vi "OAT Orbit Plot (Filtered).vi"(0 "magnitudes":T5(array[cluster]) {"magnitude" format="%.2f"; "time/rev/rpm" format="%.2f"}, 1 "orbit plot ref":refnum<vi>, 2 "reset? (F)":bool, 3 "order to display":dbl=1.0 format="%.2f", 5 "phases [phase lag]":cluster{"time/rev/rpm":dbl[], "phase":dbl[]}[](array[cluster]) {"phase" format="%.2f"; "time/rev/rpm" format="%.2f"}, 7 "magnitude/phase position info":T1, 9 "revolutions to display [rev]":cluster{"start":dbl, "duration":dbl}={"start"=0.0, "duration"=1.0} {"duration" format="%.2f"; "start" format="%.2f"}, 11 "error in (no error)":errorcluster, 12 "channel settings":T2={"shaft rotating direction"=0, "probe angles [deg]"={"X"=0, "Y"=90}} {"probe angles [deg]"."Y" max=360 step=1; "probe angles [deg]"."X" max=360 step=1; "shaft rotating direction" items=["CCW", "CW"]}, 13 "view info":T4={"dB on? (F)"=FALSE, "unwrap phase? (T)"=TRUE, "unit in degree? (T)"=TRUE}, 14 "samples/rev wanted":i32=64) -> (4 "orbit plot":T3, 10 "orbit precession direction":u16(ring) items=["forward", "backward"], 15 "error out":errorcluster)   [LabVIEW 2017]
doc: "Draws an orbit plot with unfiltered or filtered data on an XY graph. The unfiltered data comes from the <B>even-angle signals</B> input, and the filtered data comes from the <B>magnitudes</B> and <B>phases [phase lag]</B> inputs."
uses:
  <vilib>/addons/Sound and Vibration/Order Analysis/Backward Compatibility/SubVIs/oa_Orbit Plot Control.ctl
  <vilib>/addons/Sound and Vibration/Order Analysis/Misc/OAT Position Info.ctl
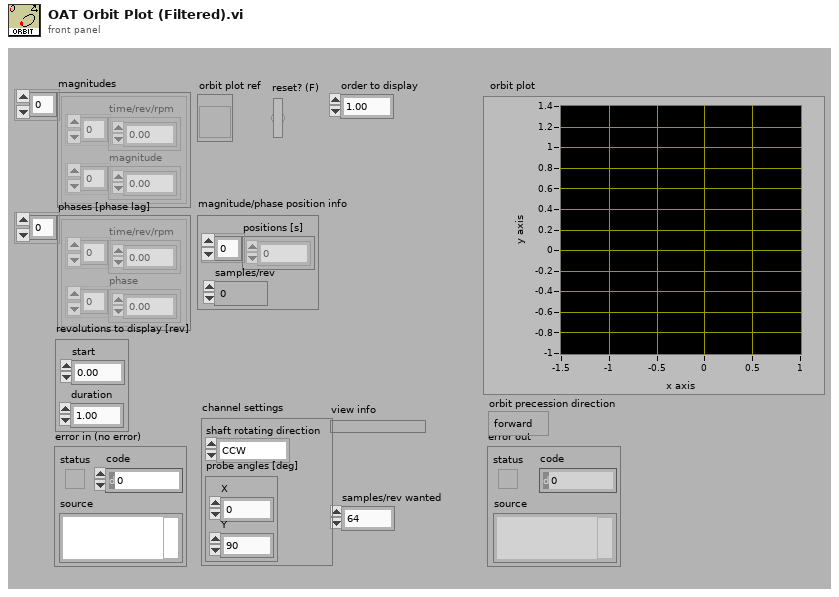
[diagram p1: front panel]
types:
  T1 = typedef "OAT Position Info.ctl" = cluster{"positions [s]":dbl[], "samples/rev":dbl}
  T2 = cluster{"shaft rotating direction":u16, "probe angles [deg]":cluster{"X":u32, "Y":u32}}
  T3 = typedef "oa_Orbit Plot Control.ctl" = cluster{dbl[], dbl[]}[]
  T4 = cluster{"dB on? (F)":bool, "unwrap phase? (T)":bool, "unit in degree? (T)":bool}
  T5 = cluster{"time/rev/rpm":dbl[], "magnitude":dbl[]}[]
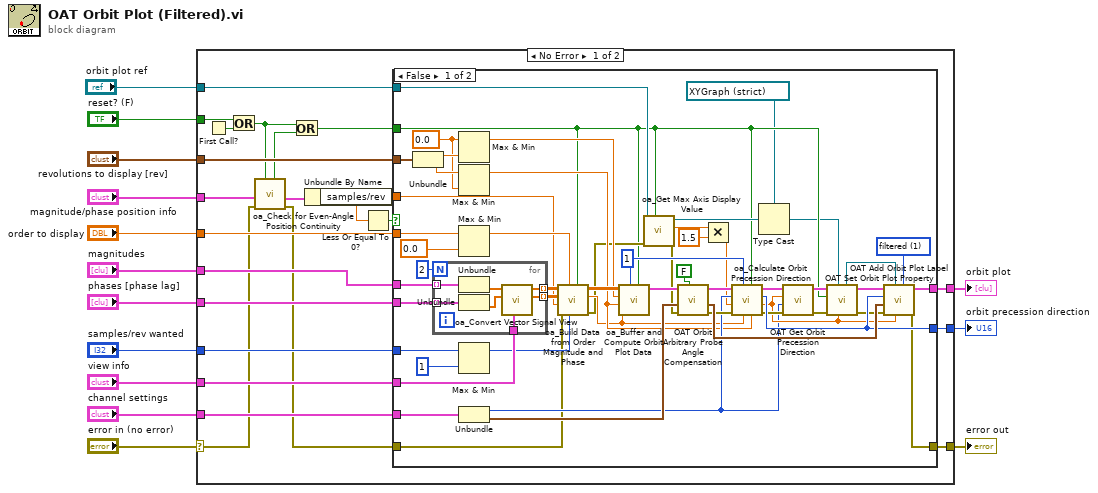
[diagram p0: block diagram]
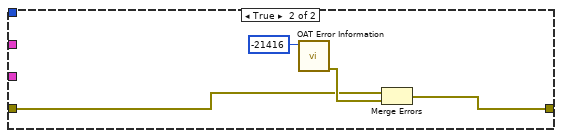
[diagram p2: hidden frame]
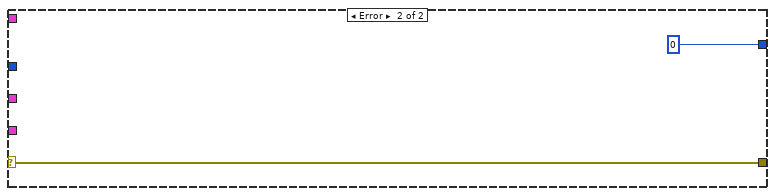
[diagram p3: hidden frame]
diagram:
  n1 = case shown="No Error" "error in (no error)" {
    selector: "error in (no error)" -> [w16 w102]
    tunnel: "order to display" -> [w27 _]
    tunnel: "magnitudes" -> [w36 _]
    tunnel: "phases [phase lag]" -> [w35 _]
    tunnel: "view info" -> [w28 _]
    tunnel: "revolutions to display [rev]" -> [w34 _]
    tunnel: [w33 _] -> w6
    tunnel: [w29 w102] -> w9
    tunnel: [w30 u16 0 ("orbit precession direction")] -> w8
    tunnel: "samples/rev wanted" -> [w32 _]
    tunnel: "channel settings" -> [w31 _]
    tunnel: "magnitude/phase position info" -> [w21 _]
    tunnel: "reset? (F)" -> [w24 _]
    tunnel: "orbit plot ref" -> [w22 _]
    frame No Error {
      n2 = First Call?() -> (First Call?: T/F=w23:bool)
      n3 = Or(x=w24, y=w23) -> (x .or. y?=w20:bool)
      n4 = call <vilib>:"oa_Check for Even-Angle Position Continuity.vi"("reset in"=w20, "error in (no error)"=w16, "even-angle position info"=w21) -> ("error out"=w15:errorcluster, "even-angle position info dup"=w17:T1, "position not continuous"=w19:bool)  [unwired: 6 in]
      n5 = Or(x=w20, y=w19) -> (x .or. y?=w18:bool)
      n6 = Unbundle By Name(w17) -> ("samples/rev"=w25:dbl)
      n7 = Less Or Equal To 0?(x=w25) -> (x <= 0?=w26:bool)
      n8 = case shown="False" w26 {
        tunnel: w36 -> [w88 _]
        tunnel: w35 -> [w87 _]
        tunnel: w34 -> [w86 _]
        tunnel: [w84 _] -> w33
        tunnel: w32 -> [w60 _]
        tunnel: w31 -> [w73 _]
        tunnel: [w71 _] -> w30
        tunnel: w15 -> [w53 w98]
        tunnel: [w68 w97] -> w29
        tunnel: w28 -> [w65 _]
        tunnel: w27 -> [w64 _]
        tunnel: w25 -> [w54 _]
        tunnel: w18 -> [w39 _]
        tunnel: w22 -> [w45 _]
        frame False {
          w74 = u16 1 items=["unfiltered", "filtered"] ("plot type")
          w51 = 1 ("tach duty")
          w82 = 0.0 ("t")
          n9 = Unbundle(w86) -> ("start"=w85:dbl, "duration"=w83:dbl)
          n10 = for {
            N: 2 -> [_]
            tunnel: w88 -> [w96] mode=indexing
            tunnel: w87 -> [w95] mode=indexing
            tunnel: w65 -> [w92]
            tunnel: [w91] -> w58 mode=indexing
            tunnel: [w90] -> w57 mode=indexing
            n11 = Unbundle(w96) -> ("magnitude"=w94:dbl[])  [unwired: 1 out]
            n12 = Unbundle(w95) -> ("phase"=w93:dbl[])  [unwired: 1 out]
            n13 = call <vilib>:"oa_Convert Vector Signal View.vi"("view"=w92, "phase"=w93, "magnitude"=w94) -> ("phase out"=w90:dbl[], "magnitude out"=w91:dbl[])  [unwired: 7 in]
          }
          n14 = Max & Min(x=w82, y=w85) -> (max(x,y)=w49:dbl)  [unwired: 1 out]
          n15 = Max & Min(x=w83, y=w82) -> (max(x,y)=w48:dbl)  [unwired: 1 out]
          n16 = Max & Min(x=w64, y=0.0 ("t")) -> (max(x,y)=w56:dbl)  [unwired: 1 out]
          n17 = Max & Min(x=w60, y=1 ("x")) -> (max(x,y)=w55:i32)  [unwired: 1 out]
          n18 = Unbundle(w73) -> ("shaft rotating direction"=w61:u16, "probe angles [deg]"=w72:cluster{"X":u32, "Y":u32})
          n19 = call <vilib>:"oa_Build Data from Order Magnitude and Phase.vi"("reset? (F)"=w39, "samples/revolution wanted"=w55, "order"=w56, "error in (no error)"=w53, "samples/revolution"=w54, "phase lag"=w57, "magnitude"=w58) -> ("error out"=w44:errorcluster, "actual samples/rev"=w47:dbl, "order waveform"=w50:dbl[][])  [unwired: 2 in]
          n20 = call <vilib>:"oa_Buffer and Compute Orbit Plot Data.vi"("reset? (F)"=w39, "tach duty"=w51, "actual samples/rev"=w47, "revolutions"=w48, "start"=w49, "order waveform"=w50) -> ("orbit data"=w52:cluster{dbl[], dbl[]}[])  [unwired: 5 in]
          n21 = call <vilib>:"oa_Get Max Axis Display Value.vi"("reset? (F)"=w39, "error in (no error)"=w44, "orbit plot ref"=w45) -> ("error out"=w43:errorcluster, "max data value out"=w41:dbl, "orbit plot out"=w46:refnum<vi>)  [unwired: 6 in]
          n22 = call <vilib>:"OAT Orbit Arbitrary Probe Angle Compensation.vi"("select methods"=FALSE, "error in (no error)"=w43, "probe angle"=w72, "XY plot data in"=w52) -> ("error out"=w67:errorcluster, "probe angle out"=w81:cluster{"X (red)":dbl, "Y (blue)":dbl}, "XY plot data out"=w79:cluster{dbl[], dbl[]}[])  [unwired: 5 in]
          n23 = Multiply(x=w41, y=1.5) -> (x*y=w42:dbl)
          n24 = call <vilib>:"oa_Calculate Orbit Precession Direction.vi"("revolutions"=w48, "reset? (F)"=w39, "actual samples/rev"=w47, "tach duty"=w51, "error in (no error)"=w67, "max axis value"=w42, "shaft rotating direction"=w61, "XY plot data in"=w79) -> ("error out"=w66:errorcluster, "max value"=w62:dbl, "orbit precession direction"=w71:u16, "XY plot data out"=w78:cluster{dbl[], dbl[]}[])
          n25 = Type Cast(type=refnum<vi> refnum ("orbit plot ref"), x=w46) -> (*(type *) &x=w38:refnum<vi>)
          n26 = call <vilib>:"OAT Get Orbit Precession Direction.vi"("error in (no error)"=w66, "shaft rotating direction"=w61, "max data value"=w62, "XY plot data in"=w78) -> ("error out"=w70:errorcluster, "XY plot data out"=w77:cluster{dbl[], dbl[]}[])  [unwired: 6 in]
          n27 = call <vilib>:"OAT Set Orbit Plot Property.vi"("max value"=w62, "orbit plot ref"=w38, "error in (no error)"=w70, "reset? (F)"=w39, "XY plot data in"=w77) -> ("error out"=w69:errorcluster, "XY plot data out"=w76:cluster{dbl[], dbl[]}[], "orbit plot ref"=w75:refnum<vi>)  [unwired: 4 in]
          n28 = call <vilib>:"OAT Add Orbit Plot Label.vi"("plot type"=w74, "max value"=w62, "orbit plot ref"=w75, "error in (no error)"=w69, "probe angle out"=w81, "orbit precession direction"=w71, "XY plot data in"=w76) -> ("error out"=w68:errorcluster, "XY plot data out"=w84:cluster{dbl[], dbl[]}[])  [unwired: 3 in]
        }
        frame True {
          n29 = call <vilib>:"OAT Error Information.vi"("error code"=-21416) -> ("error out"=w99:errorcluster)  [unwired: 6 in]
          n30 = Merge Errors(w98, w99) -> (w97:errorcluster)
        }
      }
    }
    frame Error {
    }
  }
  "error out" <- w9
  "orbit precession direction" <- w8
  "orbit plot" <- w6
